vi "Indexed Color To True Color Image.vi"(8 "error in (no error)":errorcluster, 11 "Indexed Image":T1) -> (0 "error out":errorcluster, 3 "True Color Image":T1)   [LabVIEW 2020, in "G-Image.lvlib"]
doc: "Converts an 8-bit indexed color image to a 24-bit RGB image, or a 32-bit ARGB image if the input image has a mask.\n\nNon 8-bit images are unchanged."
uses:
  G-Image.lvlib
  <vilib>/picture/picture.llb/imagedata.ctl
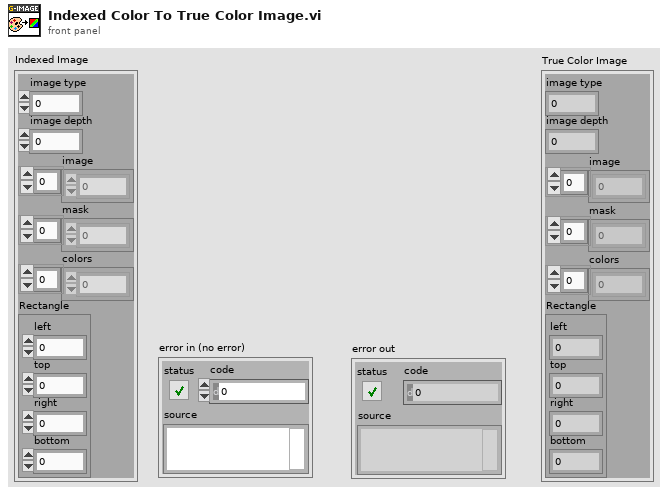
[diagram p1: front panel]
types:
  T1 = typedef "imagedata.ctl" = cluster{"image type":i32, "image depth":i32, "image":u8[], "mask":u8[], "colors":u32[], "Rectangle":cluster{"left":i16, "top":i16, "right":i16, "bottom":i16}}
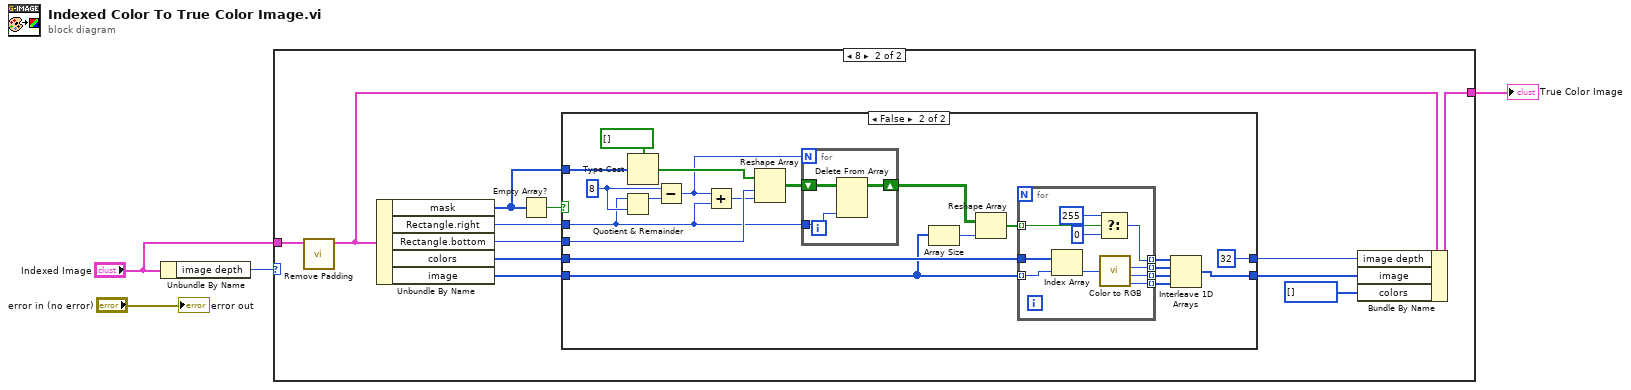
[diagram p0: block diagram]
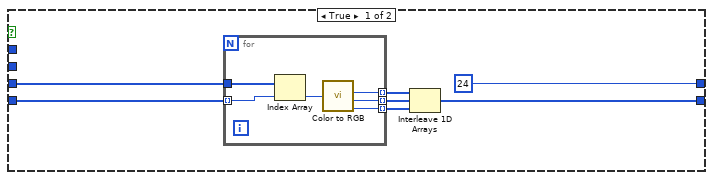
[diagram p3: hidden frame]
diagram:
  n1 = Unbundle By Name("Indexed Image") -> ("image depth"=w3:i32)
  n2 = case shown="8" w3 {
    tunnel: [w5 w10] -> w1
    tunnel: "Indexed Image" -> [w5 w14]
    frame Default {
    }
    frame 8 {
      n3 = call "Remove Padding.vi"("Image"=w14) -> ("Image Out"=w6:T1)  [unwired: 9 in, 1 out]
      n4 = Unbundle By Name(w6) -> ("mask"=w7:u8[], "Rectangle.right"=w9:i16, "Rectangle.bottom"=w8:i16, "colors"=w15:u32[], "image"=w16:u8[])
      n5 = Empty Array?(array=w7) -> (empty?=w17:bool)
      n6 = case shown="False" w17 {
        tunnel: w16 -> [w24 w42]
        tunnel: w15 -> [w23 w51]
        tunnel: w7 -> [_ w44]
        tunnel: [24 32] -> w13
        tunnel: [w19 w47] -> w12
        tunnel: w9 -> [_ w33]
        tunnel: w8 -> [_ w36]
        frame True {
          n7 = for {
            tunnel: w24 -> [w29] mode=indexing
            tunnel: w23 -> [w30]
            tunnel: [w27] -> w22 mode=indexing
            tunnel: [w26] -> w21 mode=indexing
            tunnel: [w25] -> w20 mode=indexing
            n8 = Index Array(array=w30, index=w29) -> (element=w28:u32)
            n9 = call <vilib>:"Color to RGB.vi"("Color"=w28) -> ("R"=w27:u8, "G"=w26:u8, "B"=w25:u8)  [unwired: 1 out]
          }
          n10 = Interleave 1D Arrays(w22, w21, w20) -> (w19:u8[])
        }
        frame False {
          w35 = i16 8 ("y")
          n11 = Quotient & Remainder(x=w33, y=w35) -> (x-y*floor(x/y)=w34:i16)  [unwired: 1 out]
          n12 = Type Cast(type=bool[] [], x=w44) -> (*(type *) &x=w41:bool[])
          n13 = Subtract(x=w35, y=w34) -> (x-y=w31:i16)
          n14 = Add(x=w31, y=w33) -> (x+y=w32:i16)
          n15 = Reshape Array(w41, w36, w32) -> (w40:bool[][])
          n16 = for {
            N: w31 -> [_]
            shift-right: [w53] -> w39
            shift-left: w40 -> [w54]
            tunnel: w33 -> [w52]
            n17 = Delete From Array(array=w54, index (col)=w52) -> (array with subset deleted=w53:bool[][])  [unwired: 2 in, 1 out]
          }
          n18 = Array Size(array=w42) -> (size(s)=w38:i32)
          n19 = Reshape Array(w39, w38) -> (w37:bool[])
          n20 = for {
            tunnel: w42 -> [w63] mode=indexing
            tunnel: w51 -> [w64]
            tunnel: [w61] -> w50 mode=indexing
            tunnel: [w60] -> w49 mode=indexing
            tunnel: [w59] -> w48 mode=indexing
            tunnel: w37 -> [w58] mode=indexing
            tunnel: [w55] -> w43 mode=indexing
            n21 = Index Array(array=w64, index=w63) -> (element=w62:u32)
            n22 = Select(t=u8 255, s=w58, f=u8 0) -> (s? t:f=w55:u8)
            n23 = call <vilib>:"Color to RGB.vi"("Color"=w62) -> ("R"=w61:u8, "G"=w60:u8, "B"=w59:u8)  [unwired: 1 out]
          }
          n24 = Interleave 1D Arrays(w43, w50, w49, w48) -> (w47:u8[])
        }
      }
      n25 = Bundle By Name(cluster=w6, "image depth"=w13, "image"=w12, "colors"=u32[] []) -> (w10:T1)
    }
  }
  "True Color Image" <- w1
  "error out" <- "error in (no error)"
